vi "Presynthesize.vi"(0 "Waveform in":refnum<class "Waveform.lvclass">, 5 "Channel in":refnum<class "Channel.lvclass">, 11 "error in (no error)":errorcluster) -> (4 "Waveform out":refnum<class "Waveform.lvclass">, 6 "Channel out":refnum<class "Channel.lvclass">, 15 "error out":errorcluster)   [LabVIEW 2015, in "Waveform.lvclass"]
uses:
  Waveform.lvclass
  Channel/Channel.lvclass
  Level/LevelUnits.ctl
  Channel/Channel.lvclass/Channel.ctl
  Level/Level.lvclass/Level.ctl
  Channel/Read Level.vi
  Level/Write Units.vi
  Level/Write Level.vi
  Channel/Write Level.vi
  Level/Level.lvclass
  Koop/KObject Class/KObject.lvclass
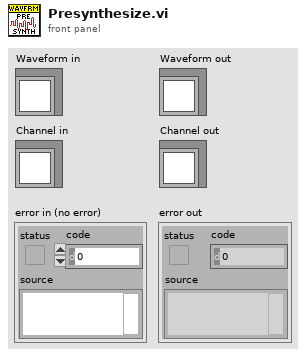
[diagram p1: front panel]
types:
  T1 = typedef "Level.lvclass/LevelUnits.ctl" = enum16{"dB atten", "dB SPL", "dB Vrms", "Volts", "dB mW", "mW", "dB HL", "dB SL"}
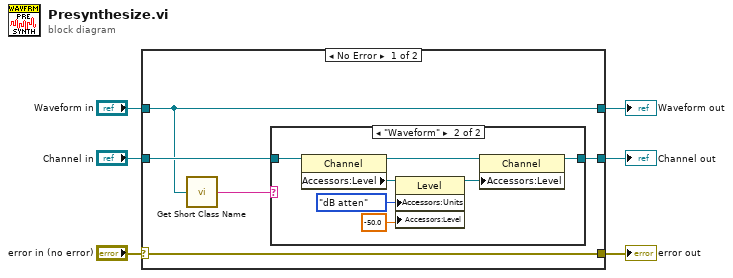
[diagram p0: block diagram]
diagram:
  n1 = case shown="No Error" "error in (no error)" {
    selector: "error in (no error)" -> [w11 w22]
    tunnel: [w11 w22] -> w5
    tunnel: [w8 w21] -> w3
    tunnel: "Waveform in" -> [w8 w21]
    tunnel: [w9 w20] -> w2
    tunnel: "Channel in" -> [w10 w20]
    frame No Error {
      n2 = call "Get Short Class Name.vi"("KObject in"=w8) -> ("Class"=w7:string)  [unwired: 4 in]
      n3 = case shown="\"Waveform\"" w7 {
        tunnel: w10 -> [w12 w19]
        tunnel: [w12 w18] -> w9
        frame "", Default {
        }
        frame "Waveform" {
          n4 = property class="Channel"(reference=w19) -> (reference out=w17:refnum<class "Channel.lvclass">, "Accessors:Level"=w16:refnum<class "Level.lvclass">)  [unwired: 1 in, 1 out]
          n5 = property class="Level"(reference=w16, "Accessors:Units"=LevelUnits."dB atten" ("Units"), "Accessors:Level"=-50.0 ("Level")) -> (reference out=w15:refnum<class "Level.lvclass">)  [unwired: 1 in, 1 out]
          n6 = property class="Channel"(reference=w17, "Accessors:Level"=w15) -> (reference out=w18:refnum<class "Channel.lvclass">)  [unwired: 1 in, 1 out]
        }
      }
    }
    frame Error {
    }
  }
  "error out" <- w5
  "Waveform out" <- w3
  "Channel out" <- w2
